vi "temperature_logger.vi"() -> (1 "temperature":dbl, 2 "time string":string, 3 "date string":string)   [LabVIEW 2017]
panel:
  in  "?":bool
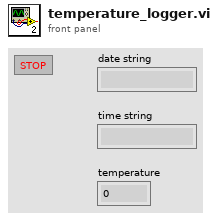
[diagram p1: front panel]
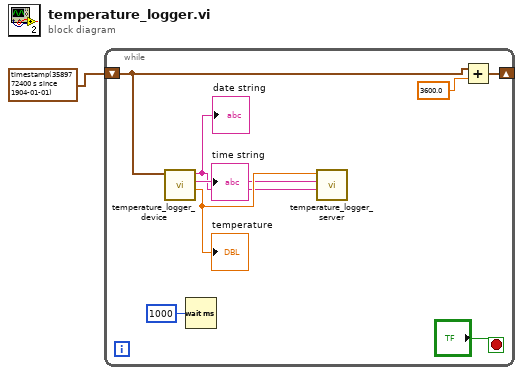
[diagram p0: block diagram]
diagram:
  n1 = while {
    shift-right: [w4] -> _
    shift-left: timestamp(3589772400 s since 1904-01-01) ("Time Stamp") -> [w6]
    stop <- "?" stop-if-true
    n2 = call "temperature_logger_device.vi"("Time Stamp"=w6) -> ("Numeric"=w9:dbl, "time string"=w8:string, "date string"=w7:string)  [unwired: 8 in]
    "date string" <- w7
    "time string" <- w8
    "temperature" <- w9
    n3 = Wait (ms)(milliseconds to wait=u32 1000) -> ()  [unwired: 1 out]
    n4 = call "temperature_logger_server.vi"("date string"=w7, "time string"=w8, "Numeric"=w9) -> ()  [unwired: 9 in]
    n5 = Add(x=w6, y=3600.0) -> (x+y=w4:timestamp)
  }
